vi "Initialize Parameter Manager.vi"(8 "error in (no error)":errorcluster, 10 "Item Ref in":u64 format="%.0x", 11 "VI Refnum":refnum<vi>) -> (0 "error out":errorcluster, 2 "Item Ref out":u64 format="%.0x", 3 "CD Parameter Manager out":refnum<class "CD Parameter Manager.lvclass">)   [LabVIEW 2019, in "CD Parameter Manager API.lvlib" / "CD Parameter Manager.lvclass"]
uses:
  CD Parameter Manager.lvclass
  CD Parameter Manager.lvclass/CD Parameter Manager.ctl
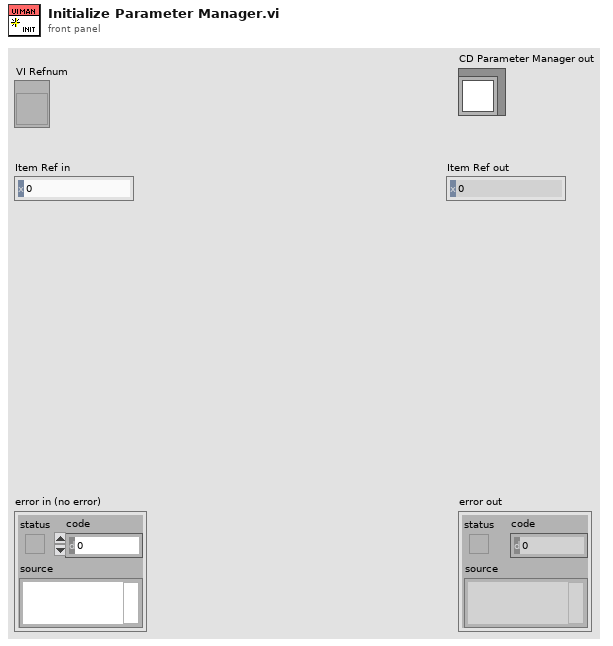
[diagram p1: front panel]
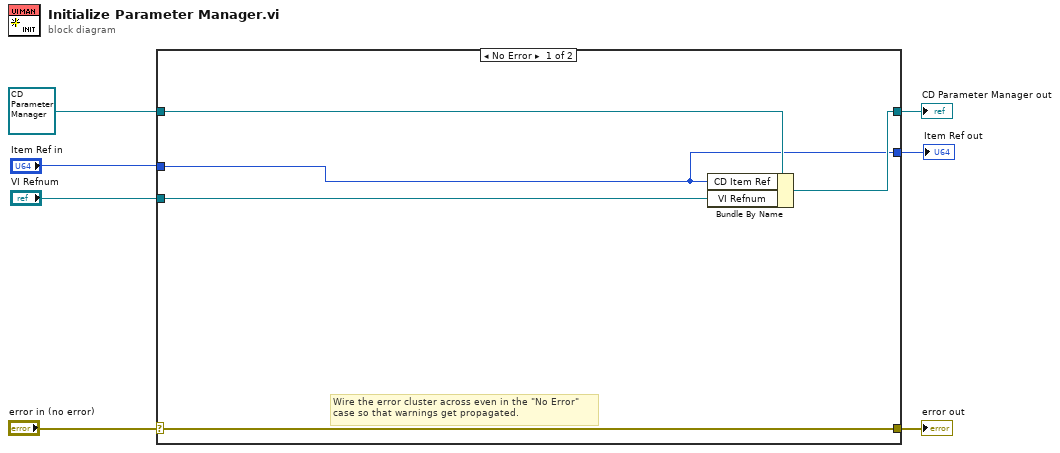
[diagram p0: block diagram]
diagram:
  n1 = case shown="No Error" "error in (no error)" {
    selector: "error in (no error)" -> [w12 w15]
    tunnel: [w12 w15] -> w6
    tunnel: [w9 w14] -> w4
    tunnel: refnum<class "CD Parameter Manager.lvclass"> refnum ("CD Parameter Manager in") -> [w11 w14]
    tunnel: "VI Refnum" -> [w10 _]
    tunnel: "Item Ref in" -> [w8 w13]
    tunnel: [w8 w13] -> w1
    frame No Error {
      # "Wire the error cluster across even in the \"No Error\"\ncase so that warnings get propagated."
      n2 = Bundle By Name(cluster=w11, "CD Item Ref"=w8, "VI Refnum"=w10) -> (w9:refnum<class "CD Parameter Manager.lvclass">)
    }
    frame Error {
    }
  }
  "error out" <- w6
  "CD Parameter Manager out" <- w4
  "Item Ref out" <- w1
